vi "CRYInsert Operator Array.vi"(4 "OpenAll/Open":bool, 6 "Front Panel Window:Window Bounds":T1, 7 "Title nID":i32, 8 "VI nID":i32, 9 "pVIRef_Out":refnum<vi>, 11 "sOperator Type":string) -> ()   [LabVIEW 2013]
uses:
  <vilib>/Utility/miscctls.llb/LVRectTypeDef.ctl
  SubVI/CRYMisc vis settings global.vi
  CRYWindow/SubVI/CRYMain Sub Window Global.vi
panel:
  out "error out":errorcluster
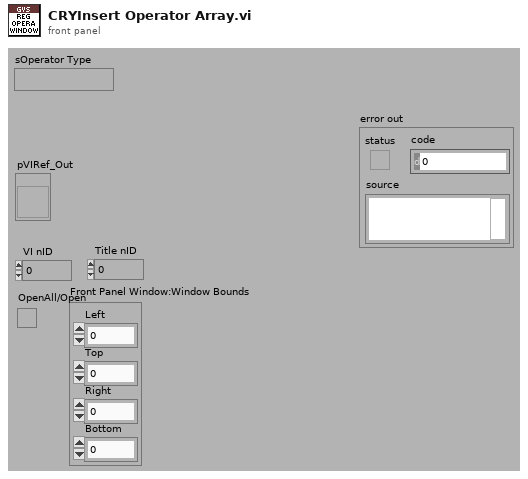
[diagram p1: front panel]
types:
  T1 = typedef "LVRectTypeDef.ctl" = cluster{"Left":i16, "Top":i16, "Right":i16, "Bottom":i16}
  T2 = cluster{"VI Ref":refnum<vi>[], "VI nID":i32[], "Title nID":i32[]}
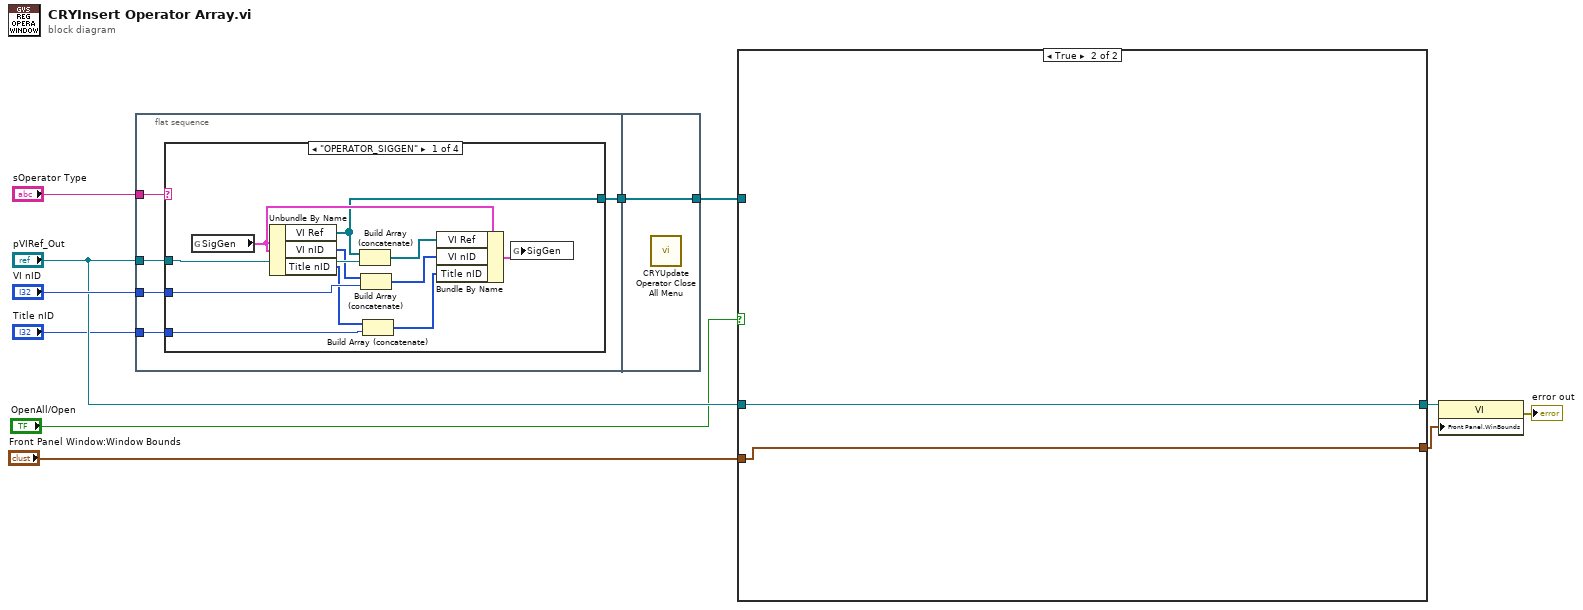
[diagram p0: block diagram]
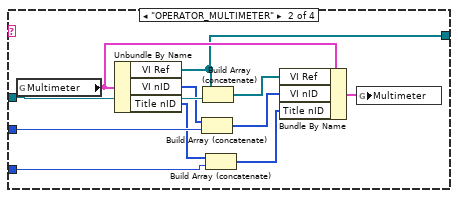
[diagram p2: hidden frame]
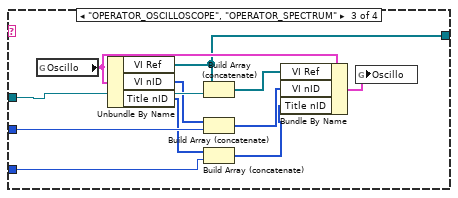
[diagram p3: hidden frame]
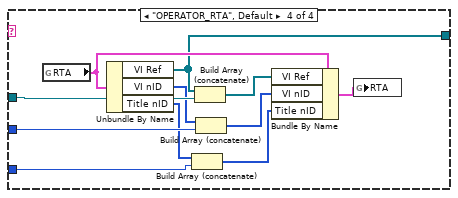
[diagram p4: hidden frame]
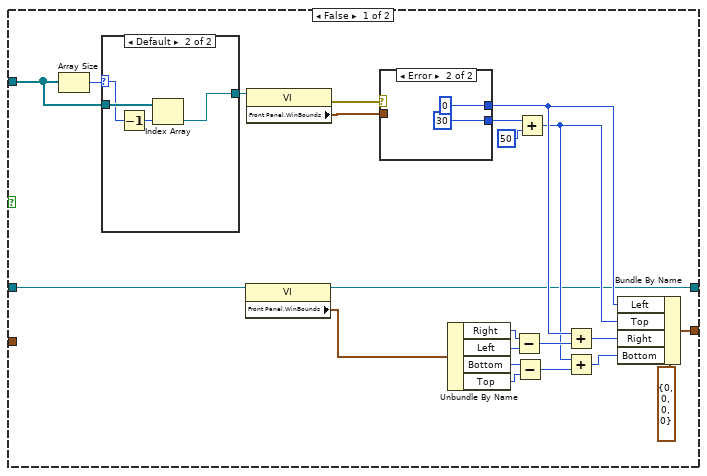
[diagram p5: hidden frame]
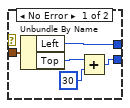
[diagram p6: hidden frame]
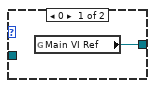
[diagram p7: hidden frame]
diagram:
  n1 = flat-sequence {
    tunnel: "sOperator Type" -> [w16]
    tunnel: "VI nID" -> [w15]
    tunnel: "pVIRef_Out" -> [w14]
    tunnel: "Title nID" -> [w12]
    tunnel: [w13] -> w1
    tunnel: [w61] -> w7
    tunnel: w1 -> [w61]
    frame #0 {
      n2 = case shown="\"OPERATOR_SIGGEN\"" w16 {
        tunnel: w14 -> [w26 w37 w48 w60]
        tunnel: w15 -> [w23 w35 w46 w57]
        tunnel: [w20 w31 w42 w53] -> w13
        tunnel: w12 -> [w18 w28 w40 w51]
        frame "OPERATOR_SIGGEN" {
          n3 = global read "CRYMisc vis settings global.vi" "SigGen"() -> (w21:T2)
          n4 = Unbundle By Name(w21) -> ("VI Ref"=w20:refnum<vi>[], "VI nID"=w25:i32[], "Title nID"=w19:i32[])
          n5 = Build Array (concatenate)(w20, w26) -> (w27:refnum<vi>[])
          n6 = Build Array (concatenate)(w25, w23) -> (w24:i32[])
          n7 = Build Array (concatenate)(w19, w18) -> (w17:i32[])
          n8 = Bundle By Name(cluster=w21, "VI Ref"=w27, "VI nID"=w24, "Title nID"=w17) -> (w22:T2)
          n9 = global write "CRYMisc vis settings global.vi" "SigGen"(w22) -> ()
        }
        frame "OPERATOR_MULTIMETER" {
          n10 = global read "CRYMisc vis settings global.vi" "Multimeter"() -> (w32:T2)
          n11 = Unbundle By Name(w32) -> ("VI Ref"=w31:refnum<vi>[], "VI nID"=w36:i32[], "Title nID"=w30:i32[])
          n12 = Build Array (concatenate)(w36, w35) -> (w34:i32[])
          n13 = Build Array (concatenate)(w31, w37) -> (w38:refnum<vi>[])
          n14 = Build Array (concatenate)(w30, w28) -> (w29:i32[])
          n15 = Bundle By Name(cluster=w32, "VI Ref"=w38, "VI nID"=w34, "Title nID"=w29) -> (w33:T2)
          n16 = global write "CRYMisc vis settings global.vi" "Multimeter"(w33) -> ()
        }
        frame "OPERATOR_OSCILLOSCOPE", "OPERATOR_SPECTRUM" {
          n17 = global read "CRYMisc vis settings global.vi" "Oscillo"() -> (w43:T2)
          n18 = Unbundle By Name(w43) -> ("VI Ref"=w42:refnum<vi>[], "VI nID"=w47:i32[], "Title nID"=w41:i32[])
          n19 = Build Array (concatenate)(w42, w48) -> (w49:refnum<vi>[])
          n20 = Build Array (concatenate)(w47, w46) -> (w45:i32[])
          n21 = Build Array (concatenate)(w41, w40) -> (w39:i32[])
          n22 = Bundle By Name(cluster=w43, "VI Ref"=w49, "VI nID"=w45, "Title nID"=w39) -> (w44:T2)
          n23 = global write "CRYMisc vis settings global.vi" "Oscillo"(w44) -> ()
        }
        frame "OPERATOR_RTA", Default {
          n24 = global read "CRYMisc vis settings global.vi" "RTA"() -> (w54:T2)
          n25 = Unbundle By Name(w54) -> ("VI Ref"=w53:refnum<vi>[], "VI nID"=w58:i32[], "Title nID"=w52:i32[])
          n26 = Build Array (concatenate)(w52, w51) -> (w50:i32[])
          n27 = Build Array (concatenate)(w53, w60) -> (w59:refnum<vi>[])
          n28 = Build Array (concatenate)(w58, w57) -> (w56:i32[])
          n29 = Bundle By Name(cluster=w54, "VI Ref"=w59, "VI nID"=w56, "Title nID"=w50) -> (w55:T2)
          n30 = global write "CRYMisc vis settings global.vi" "RTA"(w55) -> ()
        }
      }
    }
    frame #1 {
      n31 = call "CRYUpdate Operator Close All Menu.vi"() -> ()  [unwired: 12 in]
    }
  }
  n32 = case shown="True" "OpenAll/Open" {
    tunnel: "pVIRef_Out" -> [w77 w96]
    tunnel: [w75 w97] -> w8
    tunnel: w7 -> [w64 _]
    tunnel: [w63 w96] -> w6
    tunnel: "Front Panel Window:Window Bounds" -> [_ w97]
    frame False {
      n33 = Array Size(array=w64) -> (size(s)=w78:i32)
      n34 = case shown="Default" w78 {
        selector: w78 -> [_ w94]
        tunnel: [w91 w92] -> w65
        tunnel: w64 -> [_ w95]
        frame 0 {
          n35 = global read "CRYMain Sub Window Global.vi" "Main VI Ref"() -> (w91:refnum<vi>)
        }
        frame Default {
          n36 = Decrement(x=w94) -> (x-1=w93:i32)
          n37 = Index Array(array=w95, index=w93) -> (element=w92:refnum<vi>)
        }
      }
      n38 = property class="VI"(reference=w77) -> (reference out=w63:refnum<vi>, "Front Panel.WinBounds"=w83:T1)  [unwired: 1 in, 1 out]
      n39 = property class="VI"(reference=w65) -> (error out=w62:errorcluster, "Front Panel.WinBounds"=w68:T1)  [unwired: 1 in, 1 out]
      n40 = case shown="Error" w62 {
        tunnel: [w84 i16 30 ("left")] -> w69
        tunnel: w68 -> [w88 _]
        tunnel: [w87 i16 0 ("left")] -> w67
        frame No Error {
          n41 = Unbundle By Name(w88) -> ("Left"=w87:i16, "Top"=w86:i16)
          n42 = Add(x=w86, y=i16 30) -> (x+y=w84:i16)
        }
        frame Error {
        }
      }
      n43 = Unbundle By Name(w83) -> ("Right"=w82:i16, "Left"=w81:i16, "Bottom"=w80:i16, "Top"=w79:i16)
      n44 = Subtract(x=w82, y=w81) -> (x-y=w74:i16)
      n45 = Subtract(x=w80, y=w79) -> (x-y=w72:i16)
      n46 = Add(x=w69, y=i16 50) -> (x+y=w66:i16)
      n47 = Add(x=w67, y=w74) -> (x+y=w73:i16)
      n48 = Add(x=w66, y=w72) -> (x+y=w71:i16)
      n49 = Bundle By Name(cluster=T1 {"Left"=0, "Top"=0, "Right"=0, "Bottom"=0} ("Front Panel Window:Panel Bounds"), "Left"=w67, "Top"=w66, "Right"=w73, "Bottom"=w71) -> (w75:T1)
    }
    frame True {
    }
  }
  n50 = property class="VI"(reference=w6, "Front Panel.WinBounds"=w8) -> (error out=→"error out":errorcluster)  [unwired: 1 in, 1 out]
